vi "Write SP Min Usable Z.vi"(8 "error in (no error)":errorcluster, 10 "SP Min Usable Z":dbl=4500.0, 11 "SemiProbe in":refnum<class "SemiProbe.lvclass">) -> (0 "error out":errorcluster, 3 "SemiProbe out":refnum<class "SemiProbe.lvclass">)   [LabVIEW 2019, in "SemiProbe.lvclass"]
uses:
  SemiProbe.lvclass
  SemiProbe.lvclass/SemiProbe.ctl
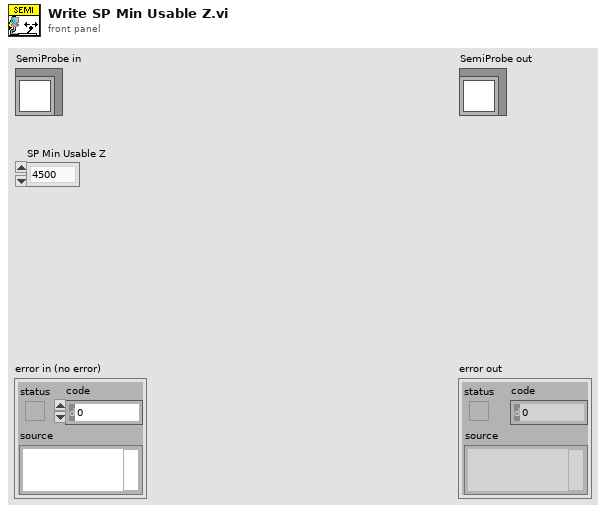
[diagram p1: front panel]
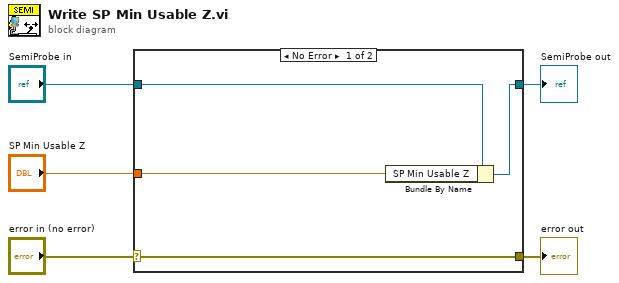
[diagram p0: block diagram]
diagram:
  n1 = case shown="No Error" "error in (no error)" {
    selector: "error in (no error)" -> [w9 w10]
    tunnel: [w9 w10] -> w4
    tunnel: [w7 w11] -> w2
    tunnel: "SemiProbe in" -> [w8 w11]
    tunnel: "SP Min Usable Z" -> [w6 _]
    frame No Error {
      n2 = Bundle By Name(cluster=w8, "SP Min Usable Z"=w6) -> (w7:refnum<class "SemiProbe.lvclass">)
    }
    frame Error {
    }
  }
  "error out" <- w4
  "SemiProbe out" <- w2
